vi "CMI ckd2 Close.vi"(8 "error in":errorcluster, 11 "session":T1) -> (0 "error out":errorcluster, 3 "session out":T1)   [LabVIEW 2020, in "AWG.lvlib"]
doc: "Closes divider interface."
uses:
  AWG.lvlib
  CMI ckd2 Session.ctl
  CMI ckd2 Source Mode.ctl
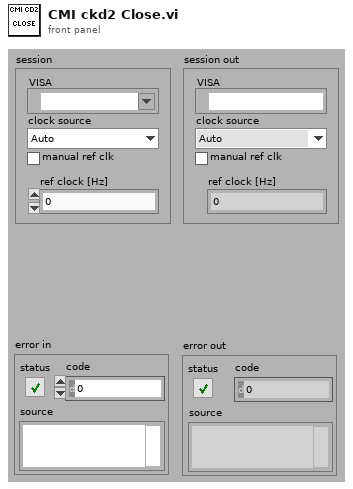
[diagram p1: front panel]
types:
  T1 = typedef "AWG.lvlib/CMI ckd2 Session.ctl" = cluster{"VISA":refnum<visa-resource-name>, "clock source":T2, "manual ref clk":bool, "ref clock [Hz]":dbl}
  T2 = typedef "AWG.lvlib/CMI ckd2 Source Mode.ctl" = enum16{"Auto", "LF clock", "HF clock", "Internal"}
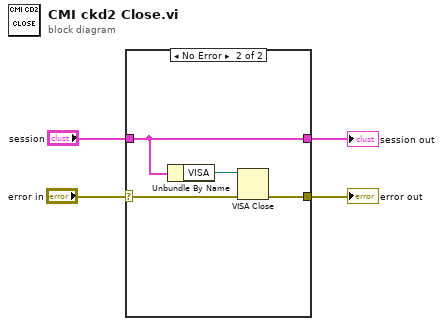
[diagram p0: block diagram]
diagram:
  n1 = case shown="No Error" "error in" {
    selector: "error in" -> [w5 w10]
    tunnel: [w6 w7] -> w2
    tunnel: [w5 w8] -> w4
    tunnel: "session" -> [w6 w7]
    frame Error {
    }
    frame No Error {
      n2 = Unbundle By Name(w7) -> ("VISA"=w9:refnum<visa-resource-name>)
      n3 = VISA Close(VISA resource name=w9, error in (no error)=w10) -> (error out=w8:errorcluster)
    }
  }
  "error out" <- w4
  "session out" <- w2
